vi "HR threshold range.vi"(8 "error in":errorcluster, 9 "HR Set":u8, 10 "Age":u8, 11 "Sex":enum16{"Male", "Female"}(ring)) -> (0 "error out":errorcluster, 2 "Range 80%":dbl, 3 "Range 60%":dbl)   [LabVIEW 2016]
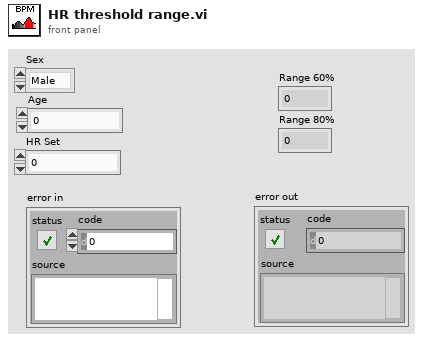
[diagram p1: front panel]
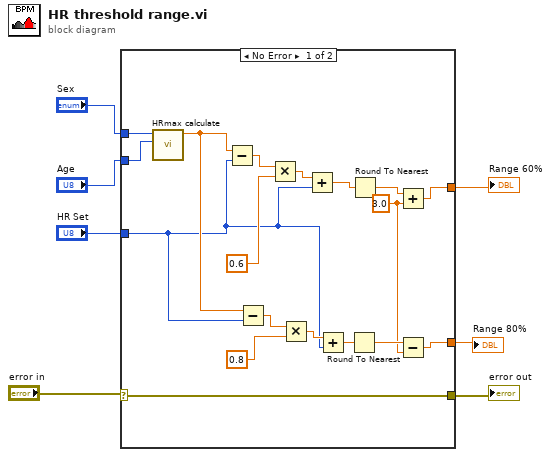
[diagram p0: block diagram]
diagram:
  n1 = case shown="No Error" "error in" {
    selector: "error in" -> [w13 w26]
    tunnel: "Sex" -> [w25 _]
    tunnel: "Age" -> [w24 _]
    tunnel: "HR Set" -> [w16 _]
    tunnel: [w11 _] -> w4
    tunnel: [w9 _] -> w3
    tunnel: [w13 w26] -> w1
    frame No Error {
      w8 = 3.0 ("y")
      n2 = call "HRmax calculate.vi"("Age"=w24, "Sex"=w25) -> ("HR Max"=w17:dbl)  [unwired: 8 in, 1 out]
      n3 = Subtract(x=w17, y=w16) -> (x-y=w23:dbl)
      n4 = Subtract(x=w17, y=w16) -> (x-y=w19:dbl)
      n5 = Multiply(x=w23, y=0.6) -> (x*y=w21:dbl)
      n6 = Multiply(x=w19, y=0.8) -> (x*y=w20:dbl)
      n7 = Add(x=w21, y=w16) -> (x+y=w15:dbl)
      n8 = Add(x=w20, y=w16) -> (x+y=w14:dbl)
      n9 = Round To Nearest(number=w14) -> (nearest integer value=w10:dbl)
      n10 = Round To Nearest(number=w15) -> (nearest integer value=w12:dbl)
      n11 = Add(x=w12, y=w8) -> (x+y=w11:dbl)
      n12 = Subtract(x=w10, y=w8) -> (x-y=w9:dbl)
    }
    frame Error {
    }
  }
  "Range 60%" <- w4
  "Range 80%" <- w3
  "error out" <- w1
